vi "LM35_Thermostat_with_Hysteresis.vi"() -> ()   [LabVIEW 2021]
uses:
  <vilib>/Utility/error.llb/DialogType.ctl
  <vilib>/Instr/_visa.llb/VISA Configure Serial Port (Instr).vi
panel:
  out "FAN STATUS":bool
  out "HEATER STATUS":bool
  out "read buffer":string="\r\n"
  in  "STOP":bool
  in  "VISA resource name":refnum<visa-resource-name>="COM4"
  out "Waveform Chart":cluster{dbl, dbl, dbl}(graph)={24.4, 27.4, 23.4}
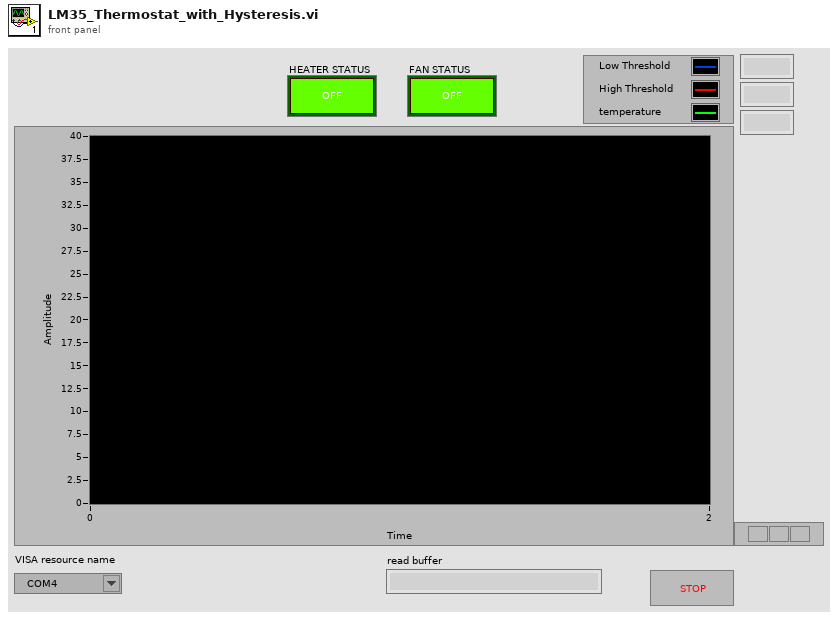
[diagram p1: front panel]
types:
  T1 = typedef "DialogType.ctl" = u16
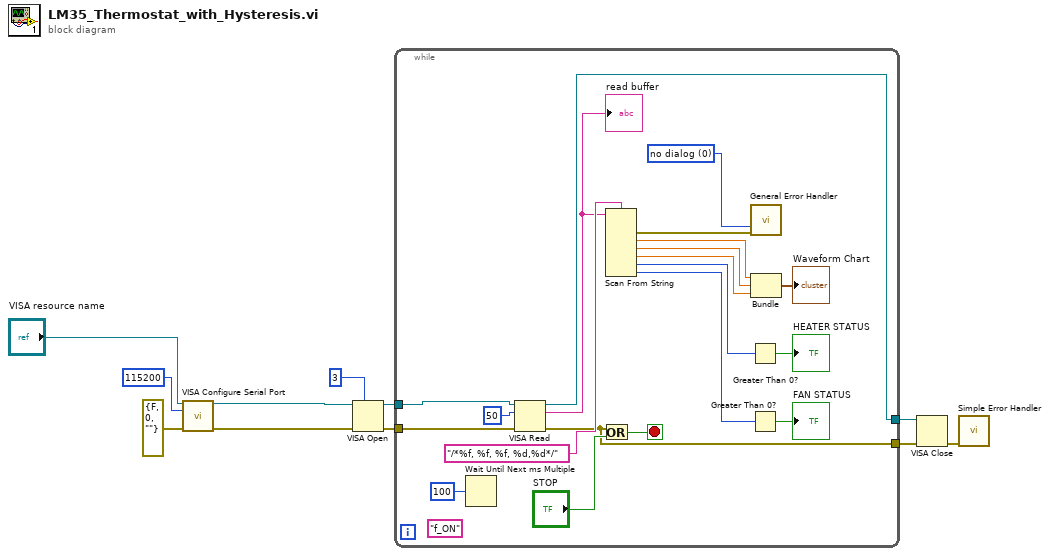
[diagram p0: block diagram]
diagram:
  n1 = call-poly "VISA Configure Serial Port"("VISA resource name"="VISA resource name", "baud rate (9600)"=u32 115200, "error in (no error)"=errorcluster {"status"=FALSE, "code"=0, "source"=""}) -> ("VISA resource name out"=w9:refnum<visa-resource-name>, "error out"=w10:errorcluster)  [unwired: 11 in]
  n2 = VISA Open(timeout (0)=u32 3 ("VISA Open timeout (0)"), error in (no error)=w10, VISA resource name=w9) -> (VISA resource name=w2:refnum<visa-resource-name>, error out=w1:errorcluster)  [unwired: 2 in]
  n3 = while {
    tunnel: w2 -> [w31]
    tunnel: [w27] -> w6
    tunnel: w1 -> [w30]
    tunnel: [w19] -> w8
    stop <- w29 stop-if-true
    (unwired) "f_ON" ("y")
    w17 = T1 0 items=["no dialog", "OK message", "continue or stop message", "OK message + warnings", "continue/stop + warnings"] ("type of dialog (OK msg:1)")
    n4 = Wait Until Next ms Multiple(millisecond multiple=u32 100) -> ()  [unwired: 1 out]
    n5 = VISA Read(VISA resource name=w31, byte count=u32 50, error in (no error)=w30) -> (VISA resource name out=w27:refnum<visa-resource-name>, read buffer=w16:string, error out=w19:errorcluster)  [unwired: 1 out]
    "read buffer" <- w16
    n6 = Or(x=w19, y="STOP") -> (x .or. y?=w29:bool)
    n7 = Scan From String "Scan From String"(format string="/*%f, %f, %f, %d,%d*/", input string=w16) -> (error out=w18:errorcluster, output 1=w25:dbl, output 2=w24:dbl, output 3=w23:dbl, output 4=w13:i32, output 5=w12:i32)  [unwired: 7 in, 2 out]
    n8 = Greater Than 0?(x=w13) -> (x > 0?=→"HEATER STATUS":bool)
    n9 = Greater Than 0?(x=w12) -> (x > 0?=→"FAN STATUS":bool)
    n10 = call <vilib>:"General Error Handler.vi"("type of dialog (OK msg:1)"=w17, "error in (no error)"=w18) -> ()  [unwired: 9 in, 5 out]
    n11 = Bundle(w25, w24, w23) -> (→"Waveform Chart":cluster{dbl, dbl, dbl})  [unwired: 1 in]
  }
  n12 = VISA Close(VISA resource name=w6, error in (no error)=w8) -> (error out=w7:errorcluster)
  n13 = call <vilib>:"Simple Error Handler.vi"("error in (no error)"=w7) -> ()  [unwired: 4 in, 5 out]
